vi "Read Alarm Status.vi"(7 "Unit Address (1)":i16=1, 8 "error in (no error)":errorcluster {"code" format="%.0x"}, 10 "Alarm Output (1)":i16=1, 11 "VISA resource name":refnum<visa-resource-name>) -> (0 "error out":errorcluster {"code" format="%.0x"}, 2 "Value":bool, 3 "VISA resource name out":refnum<visa-resource-name>)   [LabVIEW 2010]
doc: "This VI is used to read Alarm Output status."
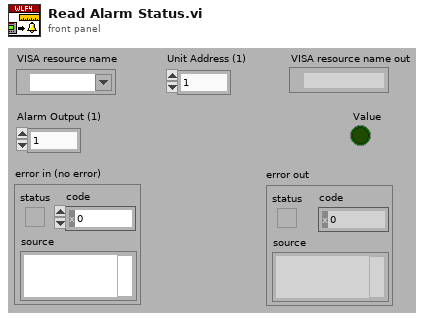
[diagram p1: front panel]
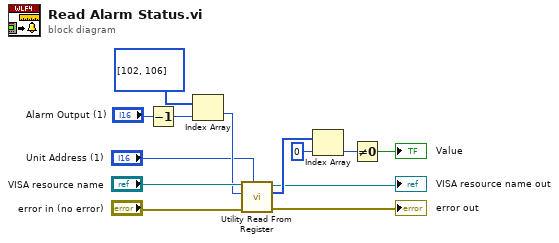
[diagram p0: block diagram]
diagram:
  n1 = Decrement(x="Alarm Output (1)") -> (x-1=w8:i16)
  n2 = Index Array(array=i32[] [102, 106], index=w8) -> (element=w9:i32)
  n3 = call "Utility Read From Register.vi"("Unit Address (1)"="Unit Address (1)", "error in (no error)"="error in (no error)", "Register Address (0)"=w9, "VISA resource name"="VISA resource name") -> ("error out"=→"error out":errorcluster, "Data"=w5:i16[], "VISA resource name out"=→"VISA resource name out":refnum<visa-resource-name>)  [unwired: 5 in]
  n4 = Index Array(array=w5, index=0) -> (element=w2:i16)
  n5 = Not Equal To 0?(x=w2) -> (x != 0?=→"Value":bool)
